vi "写入行.vi"(8 "error in (no error)":errorcluster caption="错误输入（无错误）", 10 "行数据":string, 11 "串口 输入":refnum<class "串口.lvclass"> caption="DNL_LabVIEW Object in") -> (0 "error out":errorcluster caption="错误输出", 3 "串口 输出":refnum<class "串口.lvclass"> caption="DNL_LabVIEW Object out")   [LabVIEW 2012, in "串口.lvclass"]
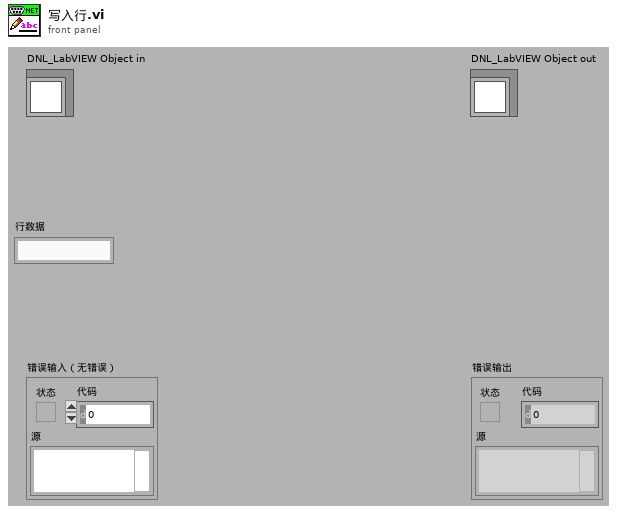
[diagram p1: front panel]
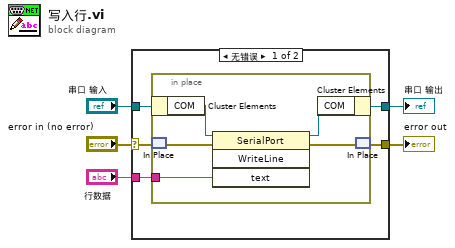
[diagram p0: block diagram]
diagram:
  n1 = case shown="无错误" "error in (no error)" {
    selector: "error in (no error)" -> [w8 w17]
    tunnel: [w7 w17] -> w4
    tunnel: [w6 w16] -> w2
    tunnel: "串口 输入" -> [w10 w16]
    tunnel: "行数据" -> [w9 _]
    frame No Error {
      n2 = in-place {
        in-place-border: w9 -> [w14]
        n3 = in-place-cluster #1(w10) -> ("COM"=w15:refnum<k24>)
        n4 = in-place-match #2(w8) -> (w13:errorcluster)
        n5 = invoke class="SerialPort" method="WriteLine"(reference=w15, error in=w13, "text"=w14) -> (reference out=w11:refnum<k24>, error out=w12:errorcluster)  [unwired: 1 in, 2 out]
        n6 = in-place-cluster #1("COM"=w11) -> (w6:refnum<class "串口.lvclass">)
        n7 = in-place-match #2(w12) -> (w7:errorcluster)
      }
    }
    frame Error {
    }
  }
  "error out" <- w4
  "串口 输出" <- w2
